vi "list all types.vi"() -> (3 "all types":T1[](array[typedef]))   [LabVIEW 2013, in "tag bus.lvlib" / "tag descriptor.lvclass"]
doc: "A helper function which provides an array of all types supported in the framework."
uses:
  tag descriptor.lvclass
  Data Type.ctl
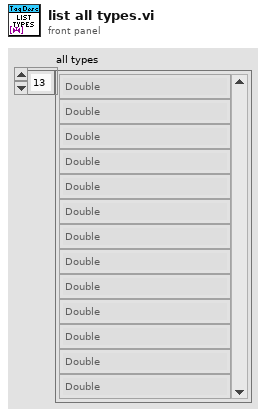
[diagram p1: front panel]
types:
  T1 = typedef "tag bus.lvlib/tag descriptor.lvclass/Data Type.ctl" = enum16{"Double", "Single", "I64", "I32", "I16", "I8", "U64", "U32", "U16", "U8", "Boolean", "String", "Array of Double", "Array of Single", "Array of I64", "Array of I32", "Array of I16", "Array of I8", "Array of U64", "Array of U32", "Array of U16", "Array of U8", "Array of Boolean", "Array of String"}
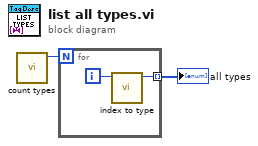
[diagram p0: block diagram]
diagram:
  n1 = call "count types.vi"() -> ("type count"=w1:i32)  [unwired: 11 in]
  n2 = for {
    N: w1 -> [_]
    tunnel: [w4] -> w2 mode=indexing
    i -> [w3]
    n3 = call "index to type.vi"("I32"=w3) -> ("type"=w4:T1)  [unwired: 10 in]
  }
  "all types" <- w2
